vi "Const Lang Default English.vi"() -> (3 "UI Descriptions":T1={"Main Panel"={"Title"={"Frame Num"={"Name"="Frame Num", "Tip"="", "Description"=""}, "Name"={"Name"="Name", "Tip"="", "Description"=""}}, "Frame Basic"={"pic"={"Name"="pic", "Tip"="", "Description"=""}, "state"={"Name"="state", "Tip"="", "Description"=""}, "wait"={"Name"="wait", "Tip"="", "Description"=""}, "next"={"Name"="next", "Tip"="Next frame number", "Description"="Next frame number  \n999: Return to frame number 0  \n1000: Remove object  \n12XX: Invisible, where XX represents the duration  \nA minus sign indicates direction reversal"}, "dvx"={"Name"="dvx", "Tip"="movement speed", "Description"="Forward (positive) and backward (negative) movement speed"}, "dvy"={"Name"="dvy", "Tip"="movement speed", "Description"="Upward (negative) and downward (positive) movement speed"}, "dvz"={"Name"="dvz", "Tip"="movement speed", "Description"="Vertical movement speed, with the direction determined by the ◆ and □ arrow keys"}, "centerx"={"Name"="centerx", "Tip"="X-axis position of the frame center", "Description"="X-axis position of the frame center (shadow), with direction from left to right"}, "centery"={"Name"="centery", "Tip"="Y-axis position of the frame center", "Description"="Y-axis position of the frame center (shadow), with direction from top to bottom"}, "sound"={"Name"="sound", "Tip"="", "Description"=""}}, "Frame Skill"={"mp"={"Name"="mp", "Tip"="HP/MP Consumption", "Description"="HP/MP Consumption  \nOOXXX: OO represents the tens digit of HP consumption, XXX represents MP consumption  \n100: Consumes 100 MP  \n4300: Consumes 40 HP and 300 MP  \n\nWhen entering a frame using hit_XX:  \n  - Positive values indicate consumption  \n  - Negative values indicate recovery  \n\nWhen entering a frame using next:  \n  - Positive values have no effect  \n  - Negative values indicate consumption"}, "hit_a"={"Name"="hit_a", "Tip"="When pressing Attack, jump to the corresponding frame number", "Description"="When pressing Attack, jump to the corresponding frame number"}, "hit_d"={"Name"="hit_d", "Tip"="When pressing Defense, jump to the corresponding frame number", "Description"="When pressing Defense, jump to the corresponding frame number"}, "hit_j"={"Name"="hit_j", "Tip"="When pressing Jump, jump to the corresponding frame number", "Description"="When pressing Jump, jump to the corresponding frame number"}, "hit_Fa"={"Name"="hit_Fa", "Tip"="When pressing Defense △ Attack, jump to the corresponding frame number", "Description"="When pressing Defense △ Attack, jump to the corresponding frame number"}, "hit_Ua"={"Name"="hit_Ua", "Tip"="When pressing Defense ◆ Attack, jump to the corresponding frame number", "Description"="When pressing Defense ◆ Attack, jump to the corresponding frame number"}, "hit_Da"={"Name"="hit_Da", "Tip"="When pressing Defense □ Attack, jump to the corresponding frame number", "Description"="When pressing Defense □ Attack, jump to the corresponding frame number"}, "hit_Fj"={"Name"="hit_Fj", "Tip"="When pressing Defense △ Jump, jump to the corresponding frame number", "Description"="When pressing Defense △ Jump, jump to the corresponding frame number"}, "hit_Uj"={"Name"="hit_Uj", "Tip"="When pressing Defense ◆ Jump, jump to the corresponding frame number", "Description"="When pressing Defense ◆ Jump, jump to the corresponding frame number"}, "hit_Dj"={"Name"="hit_Dj", "Tip"="When pressing Defense □ Jump, jump to the corresponding frame number", "Description"="When pressing Defense □ Jump, jump to the corresponding frame number"}, "hit_ja"={"Name"="hit_ja", "Tip"="When pressing Defense + Jump + Attack, jump to the corresponding frame number", "Description"="When pressing Defense + Jump + Attack, jump to the corresponding frame number"}}, "bp"={"x"={"Name"="x", "Tip"="X-axis position of mouth bleeding", "Description"="X-axis position of mouth bleeding\nBleeding occurs when HP is less than 1/3"}, "y"={"Name"="y", "Tip"="Y-axis position of mouth bleeding", "Description"="Y-axis position of mouth bleeding\nBleeding occurs when HP is less than 1/3"}}, "w"={"kind"={"Name"="kind", "Tip"="Weapon state\n1: Held in hand  \n2: Held in hand  \n3: Dropped", "Description"="Weapon state\n1: Held in hand  \n2: Held in hand  \n3: Dropped"}, "x"={"Name"="x", "Tip"="X-axis position of the weapon", "Description"="X-axis position of the weapon"}, "y"={"Name"="y", "Tip"="Y-axis position of the weapon", "Description"="Y-axis position of the weapon"}, "weaponact"={"Name"="weaponact", "Tip"="Weapon frame number\nIf outside 20~35, the weapon can be hit", "Description"="Weapon frame number\nIf outside 20~35, the weapon can be hit"}, "cover"={"Name"="cover", "Tip"="0: Weapon in front (overlays the character image)  \n1: Weapon behind (character overlays the weapon image)", "Description"="0: Weapon in front (overlays the character image)  \n1: Weapon behind (character overlays the weapon image)"}, "dvx"={"Name"="dvx", "Tip"="movement speed", "Description"="Forward (positive) and backward (negative) movement speed"}, "dvy"={"Name"="dvy", "Tip"="movement speed", "Description"="Upward (negative) and downward (positive) movement speed"}, "dvz"={"Name"="dvz", "Tip"="movement speed", "Description"="Vertical movement speed, with the direction determined by the ◆ and □ arrow keys"}, "attacking"={"Name"="attacking", "Tip"="Attack state", "Description"="Attack state\n0: No attack  \n1: Attack while standing  \n2: Attack while jumping  \n3: Attack while running  \n4: Attack while jumping forward"}}, "b"={"kind"={"Name"="kind", "Tip"="", "Description"=""}, "x"={"Name"="x", "Tip"="X-axis position of the hitbox", "Description"="X-axis position of the hitbox"}, "y"={"Name"="y", "Tip"="Y-axis position of the hitbox", "Description"="Y-axis position of the hitbox"}, "w"={"Name"="w", "Tip"="Width of the hitbox", "Description"="Width of the hitbox"}, "h"={"Name"="h", "Tip"="Height of the hitbox", "Description"="Height of the hitbox"}, "index"={"Name"="<b> index", "Tip"="body section index", "Description"="body section index"}}, "i"={"kind"={"Name"="kind", "Tip"="Injury Effect", "Description"="Injury Effect\n0: Normal attack / effect attack  \n1: Grab a stunned opponent (state 16)  \n2: Pick up a weapon  \n3: Forced grab  \n4: Attack type when thrown by an enemy  \n5: Weapon type  \n6: If an enemy is within this range, jump to a super_punch frame  \n7: Press Attack to pick up a weapon immediately  \n8: Convert injury to healing, jump to dvx frame  \n9: Reduce HP to zero after hitting an enemy  \n10: Henry's \"Death Symphony\" effect  \n11: Henry's \"Death Symphony\" effect  \n14: Block  \n15: Float  \n16: Freeze"}, "x"={"Name"="x", "Tip"="X-axis position of the hitbox", "Description"="X-axis position of the hitbox"}, "y"={"Name"="y", "Tip"="Y-axis position of the hitbox", "Description"="Y-axis position of the hitbox"}, "w"={"Name"="w", "Tip"="Width of the hitbox", "Description"="Width of the hitbox"}, "h"={"Name"="h", "Tip"="Height of the hitbox", "Description"="Height of the hitbox"}, "zwidth"={"Name"="zwidth", "Tip"="Width of the hitbox along the Z-axis", "Description"="Width of the hitbox along the Z-axis"}, "dvx"={"Name"="dvx", "Tip"="movement speed", "Description"="Forward (positive) and backward (negative) movement speed"}, "dvy"={"Name"="dvy", "Tip"="movement speed", "Description"="Upward (negative) and downward (positive) movement speed"}, "dvz"={"Name"="dvz", "Tip"="movement speed", "Description"="Vertical movement speed, with the direction determined by the ◆ and □ arrow keys"}, "fall"={"Name"="fall", "Tip"="Knockdown value", "Description"="Knockdown value\n1: Enemy pauses briefly, but the value does not accumulate toward stun  \n25: Hitting twice will stun the enemy  \n40: First hit makes the enemy step back, second hit knocks them down  \n60: First hit stuns the enemy, second hit knocks them down  \n70: Forced knockdown  \nNegative value: Does not affect the enemy's action, but grants super armor (enemy shows no hurt animation)"}, "arest"={"Name"="arest", "Tip"="Interval for repeatedly attacking a single enemy\nForcibly disables vrest", "Description"="Interval for repeatedly attacking a single enemy\nForcibly disables vrest"}, "vrest"={"Name"="vrest", "Tip"="Interval for repeatedly attacking multiple enemies\nCannot be used simultaneously with arest\nMinimum value is 4", "Description"="Interval for repeatedly attacking multiple enemies\nCannot be used simultaneously with arest\nMinimum value is 4"}, "bdefend"={"Name"="bdefend", "Tip"="Guard break value", "Description"="Guard break value\nAccumulate up to 60 to break a defending enemy  \n60: Directly breaks guard  \n100: Ignores all defense and hits directly. Items are forcibly destroyed"}, "injury"={"Name"="injury", "Tip"="", "Description"=""}, "effect"={"Name"="effect", "Tip"="Attack special effect (only for kind:0)", "Description"="Attack special effect (only for kind:0)\n0: Fist effect  \n1: Bladed weapon effect  \n2: Fire  \n20: Fire, cannot hit ball attacks  \n21: Fire, can reflect ball attacks; when combined with state 18 (fire), it will not hit allies  \n22: Fire; if dvx is positive, attack direction is inward; if dvx is negative, attack direction is outward  \n23: Hit effect; if dvx is positive, attack direction is inward; if dvx is negative, attack direction is outward  \n3: Freeze  \n30: Freeze; cannot hit state 13 characters (frozen characters)  \n4: Only attacks objects of type: 1, 2, 3, 4, 5, 6"}, "catchingact 1"={"Name"="catchingact 1", "Tip"="Only for kind: 1 (grab stunned enemy), kind: 3 (forced grab)\nAfter grabbing an enemy, jumps to the frame number", "Description"="Only for kind: 1 (grab stunned enemy), kind: 3 (forced grab)\nAfter grabbing an enemy, jumps to the frame number"}, "catchingact 2"={"Name"="catchingact 2", "Tip"="Only for kind: 1 (grab stunned enemy), kind: 3 (forced grab)\nAfter grabbing an enemy, jumps to the frame number", "Description"="Only for kind: 1 (grab stunned enemy), kind: 3 (forced grab)\nAfter grabbing an enemy, jumps to the frame number"}, "caughtact 1"={"Name"="caughtact 1", "Tip"="Only for kind: 1 (grab stunned enemy), kind: 3 (forced grab)\nAfter grabbing an enemy, the enemy's frame number jumps to the frame number", "Description"="Only for kind: 1 (grab stunned enemy), kind: 3 (forced grab)\nAfter grabbing an enemy, jumps to the frame number"}, "caughtact 2"={"Name"="caughtact 2", "Tip"="Only for kind: 1 (grab stunned enemy), kind: 3 (forced grab)\nAfter grabbing an enemy, the enemy's frame number jumps to the frame number", "Description"="Only for kind: 1 (grab stunned enemy), kind: 3 (forced grab)\nAfter grabbing an enemy, the enemy's frame number jumps to the frame number"}, "index"={"Name"="<i> index", "Tip"="injury section index", "Description"="injury section index"}}, "o"={"kind"={"Name"="kind", "Tip"="Creation type", "Description"="Creation type\n1: Dropped  \n2: Held in hand"}, "x"={"Name"="x", "Tip"="X-axis position of the object, with direction from left to right", "Description"="X-axis position of the object, with direction from left to right"}, "y"={"Name"="y", "Tip"="Y-axis position of the object, with direction from top to bottom", "Description"="Y-axis position of the object, with direction from top to bottom"}, "action"={"Name"="action", "Tip"="Frame number of the object", "Description"="Frame number of the object"}, "dvx"={"Name"="dvx", "Tip"="movement speed", "Description"="Forward (positive) and backward (negative) movement speed of the object"}, "dvy"={"Name"="dvy", "Tip"="movement speed", "Description"="Upward (negative) and downward (positive) movement speed of the object"}, "dvz"={"Name"="dvz", "Tip"="movement speed", "Description"="Vertical movement speed of the object, with direction determined by the ◆ and □ arrow keys"}, "oid"={"Name"="oid", "Tip"="Object ID", "Description"="Object ID"}, "facing"={"Name"="facing", "Tip"="Object quantity and direction", "Description"="Object quantity and direction\nOOX: OO represents the quantity. X represents the direction, where 0 = forward, 1 = reverse"}}, "c"={"kind"={"Name"="kind", "Tip"="Grab state", "Description"="1: Grabber  \n2: Grabbed"}, "x"={"Name"="x", "Tip"="X-axis position of the grabber/grabbed", "Description"="X-axis position of the grabber/grabbed"}, "y"={"Name"="y", "Tip"="Y-axis position of the grabber/grabbed", "Description"="Y-axis position of the grabber/grabbed"}, "injury"={"Name"="injury", "Tip"="Damage\nPositive value: Causes injury with hit pause effect  \nNegative value: Causes injury without hit pause effect", "Description"="Damage\nPositive value: Causes injury with hit pause effect  \nNegative value: Causes injury without hit pause effect"}, "cover"={"Name"="cover", "Tip"="Layer order\n10: Grabbed character behind  \n11: Grabbed character in front", "Description"="Layer order\n10: Grabbed character behind  \n11: Grabbed character in front"}, "vaction"={"Name"="vaction", "Tip"="Frame number of the grabbed character", "Description"="Frame number of the grabbed character"}, "aaction"={"Name"="aaction", "Tip"="When pressing Attack, jump to the corresponding frame number", "Description"="When pressing Attack, jump to the corresponding frame number"}, "taction"={"Name"="taction", "Tip"="When pressing △ + Attack, jump to the corresponding frame number", "Description"="When pressing △ + Attack, jump to the corresponding frame number"}, "hurtable"={"Name"="hurtable", "Tip"="Whether the grabbed character can be hit by others\n0: No  \n1: Yes", "Description"="Whether the grabbed character can be hit by others\n0: No  \n1: Yes"}, "decrease"={"Name"="decrease", "Tip"="Decrement value for grab duration (negative value), total duration is 301", "Description"="Decrement value for grab duration (negative value), total duration is 301"}, "fronthurtact"={"Name"="fronthurtact", "Tip"="Jump to Frame number after being hit from the front", "Description"="Jump to Frame number after being hit from the front"}, "backhurtact"={"Name"="backhurtact", "Tip"="Jump to Frame number after being hit from the back", "Description"="Jump to Frame number after being hit from the back"}, "throwvx"={"Name"="throwvx", "Tip"="X-direction speed when thrown", "Description"="X-direction speed when thrown"}, "throwvy"={"Name"="throwvy", "Tip"="Y-direction speed when thrown", "Description"="Y-direction speed when thrown"}, "throwvz"={"Name"="throwvz", "Tip"="Z-direction speed when thrown, with direction determined by the ◆ and □ arrow keys", "Description"="Z-direction speed when thrown, with direction determined by the ◆ and □ arrow keys"}, "throwinjury"={"Name"="throwinjury", "Tip"="", "Description"=""}, "dircontrol"={"Name"="dircontrol", "Tip"="", "Description"=""}}, "Other"={"File Path"={"Name"="File Path", "Tip"="", "Description"=""}, "GoTo"={"Name"="Go to Frame", "Tip"="", "Description"=""}, "Apply Change"={"Name"="Apply Change", "Tip"="", "Description"=""}, "To Next Frame"={"Name"="To Next Frame", "Tip"="", "Description"=""}}, "Menu"={"File"={"Name"="File", "Tip"="", "Description"=""}, "Open File"={"Name"="Open File", "Tip"="", "Description"=""}, "Save File"={"Name"="Save File", "Tip"="", "Description"=""}, "Exit"={"Name"="Exit", "Tip"="", "Description"=""}, "Settings"={"Name"="Settings", "Tip"="", "Description"=""}, "Preferences"={"Name"="Preferences", "Tip"="", "Description"=""}, "Help"={"Name"="Help", "Tip"="", "Description"=""}, "Show Context Help"={"Name"="Show Context Help", "Tip"="", "Description"=""}}}, "Configuration Window"={"Tab"={"Main Page"={"Name"="Main", "Tip"="", "Description"=""}, "Image Page"={"Name"="Image", "Tip"="", "Description"=""}}, "Main"={"Language"={"Name"="Language", "Tip"="", "Description"=""}, "Save"={"Name"="Save", "Tip"="", "Description"=""}, "Cancel"={"Name"="Cancel", "Tip"="", "Description"=""}}, "Path"={"Reset"={"Name"="Reset to Steam Path", "Tip"="", "Description"=""}, "Path Data"={"Name"="_res_data Folder Path", "Tip"="", "Description"=""}, "Path Png"={"Name"="_res_pngs Folder Path", "Tip"="", "Description"=""}}, "Image"={"Center Point"={"Name"={"Name"="Center Point:", "Tip"="", "Description"=""}, "Size"={"Name"="Size", "Tip"="", "Description"=""}, "Color"={"Name"="Color", "Tip"="", "Description"=""}, "Enable"={"Name"="Enable", "Tip"="", "Description"=""}}, "bp Point"={"Name"={"Name"="<bp> Point:", "Tip"="", "Description"=""}, "Size"={"Name"="Size", "Tip"="", "Description"=""}, "Color"={"Name"="Color", "Tip"="", "Description"=""}, "Enable"={"Name"="Enable", "Tip"="", "Description"=""}}, "w Point"={"Name"={"Name"="<w> Point:", "Tip"="", "Description"=""}, "Size"={"Name"="Size", "Tip"="", "Description"=""}, "Color"={"Name"="Color", "Tip"="", "Description"=""}, "Enable"={"Name"="Enable", "Tip"="", "Description"=""}}, "b Box"={"Name"={"Name"="<b> Box:", "Tip"="", "Description"=""}, "Fill Color"={"Name"="Fill Color", "Tip"="", "Description"=""}, "Border Color"={"Name"="Border Color", "Tip"="", "Description"=""}, "Enable"={"Name"="Enable", "Tip"="", "Description"=""}}, "i Box"={"Name"={"Name"="<i> Box:", "Tip"="", "Description"=""}, "Fill Color"={"Name"="Fill Color", "Tip"="", "Description"=""}, "Border Color"={"Name"="Border Color", "Tip"="", "Description"=""}, "Enable"={"Name"="Enable", "Tip"="", "Description"=""}}, "o Point"={"Name"={"Name"="<o> Point:", "Tip"="", "Description"=""}, "Size"={"Name"="Size", "Tip"="", "Description"=""}, "Color"={"Name"="Color", "Tip"="", "Description"=""}, "Enable"={"Name"="Enable", "Tip"="", "Description"=""}}, "c Point"={"Name"={"Name"="<c> Point:", "Tip"="", "Description"=""}, "Size"={"Name"="Size", "Tip"="", "Description"=""}, "Color"={"Name"="Color", "Tip"="", "Description"=""}, "Enable"={"Name"="Enable", "Tip"="", "Description"=""}}}}})   [LabVIEW 2018, in "Framework.lvlib" / "Framework.lvclass"]
uses:
  Framework/Framework/Framework.lvclass
  Const Lang Setting.ctl
  Const UI Desc Frame Title.ctl
  Const Lang Property.ctl
  Const UI Desc Frame Basic.ctl
  Const UI Desc Frame Skill.ctl
  Const UI Desc Frame bp.ctl
  Const UI Desc Frame w.ctl
  Const UI Desc Frame b.ctl
  Const UI Desc Frame i.ctl
  Const UI Desc Frame o.ctl
  Const UI Desc Frame c.ctl
  Const UI Desc Other.ctl
  Const UI Desc Menu.ctl
  Const Lang CfgWnd Tab.ctl
  Const Lang CfgWnd Main.ctl
  Const Lang CfgWnd Path.ctl
  Framework/Framework/Const Lang CfgWnd Image.ctl
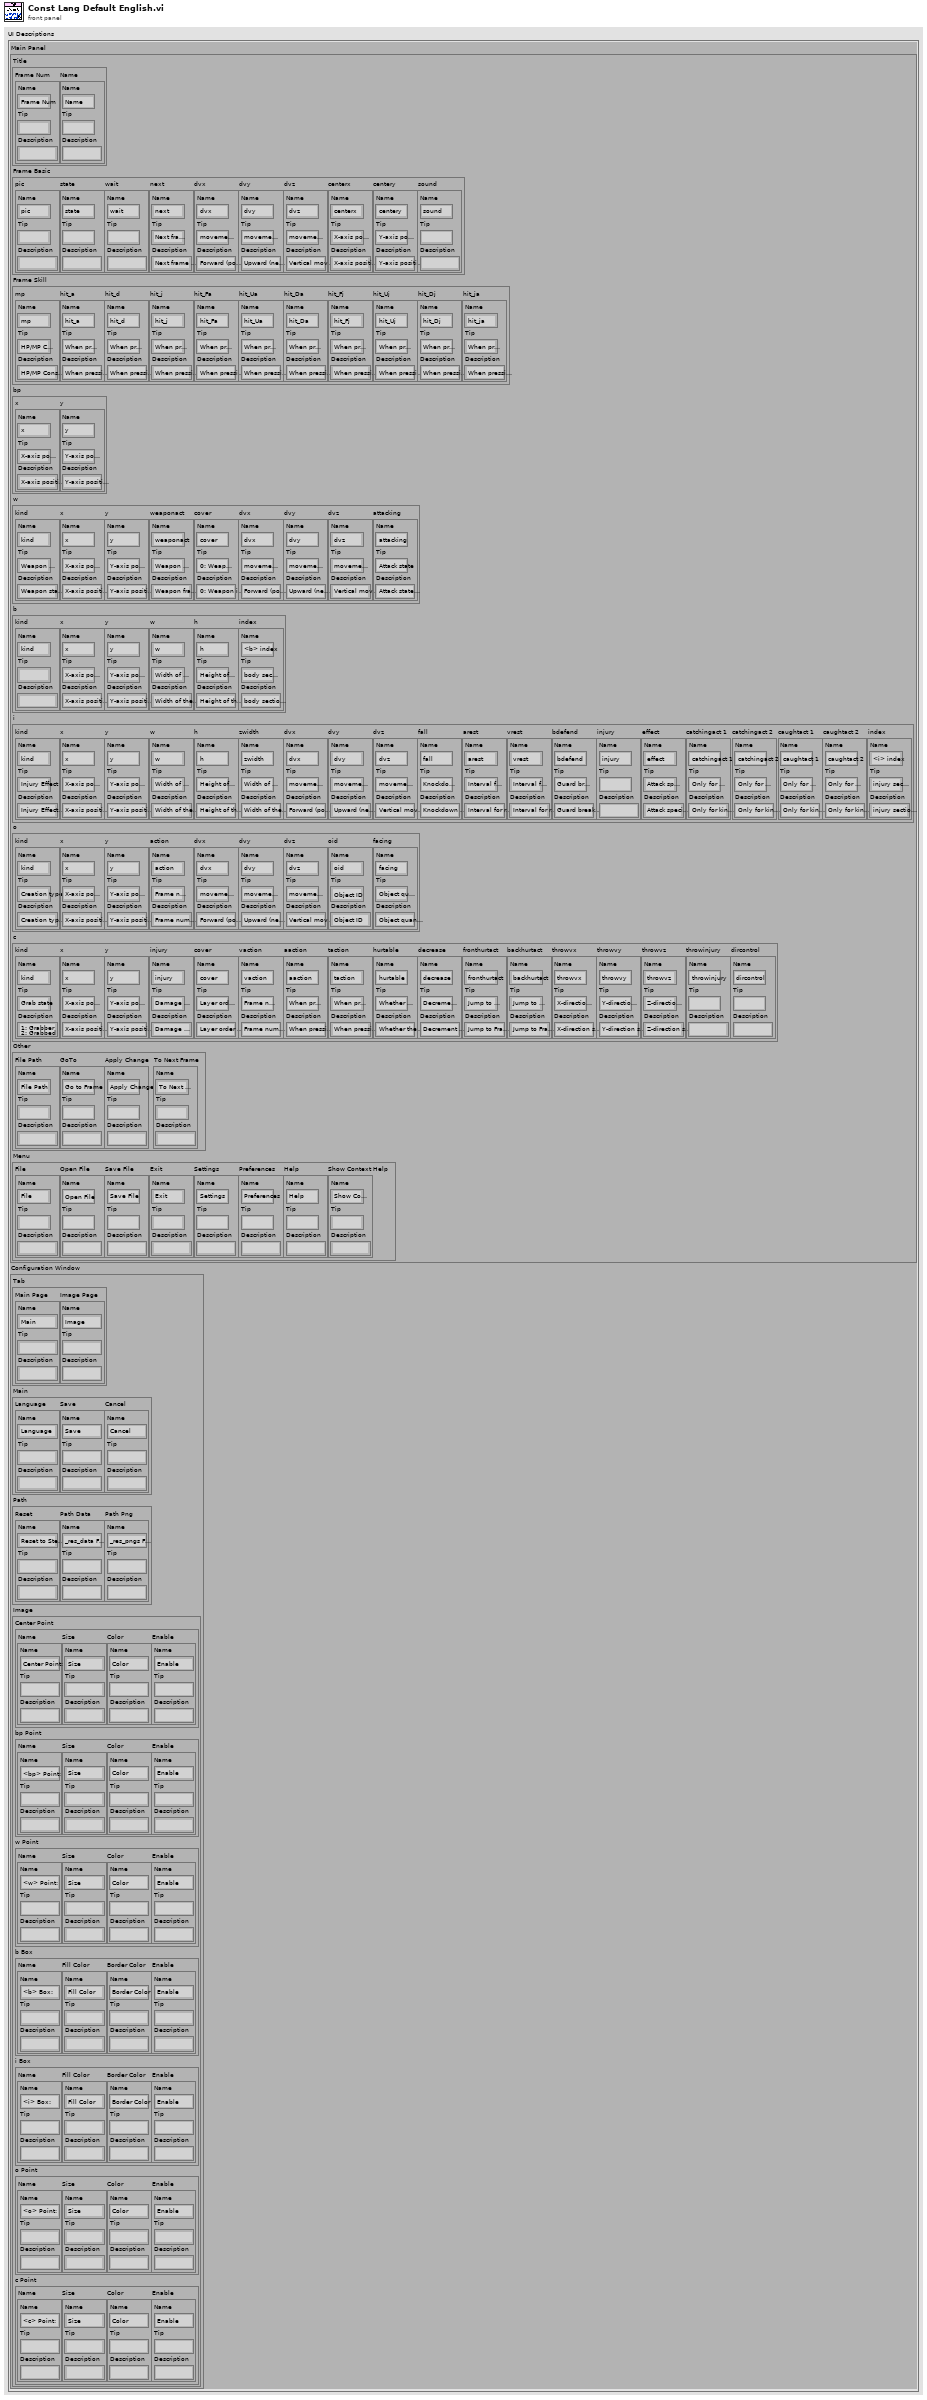
[diagram p1: front panel]
types:
  T1 = typedef "Framework.lvlib/Framework.lvclass/Const Lang Setting.ctl" = cluster{"Main Panel":cluster{"Title":T2, "Frame Basic":T4, "Frame Skill":T5, "bp":T6, "w":T7, "b":T8, "i":T9, "o":T10, "c":T11, "Other":T12, "Menu":T13}, "Configuration Window":cluster{"Tab":T14, "Main":T15, "Path":T16, "Image":T17}}
  T2 = typedef "Framework.lvlib/Framework.lvclass/Const UI Desc Frame Title.ctl" = cluster{"Frame Num":T3, "Name":T3}
  T3 = typedef "Framework.lvlib/Framework.lvclass/Const Lang Property.ctl" = cluster{"Name":string, "Tip":string, "Description":string}
  T4 = typedef "Framework.lvlib/Framework.lvclass/Const UI Desc Frame Basic.ctl" = cluster{"pic":T3, "state":T3, "wait":T3, "next":T3, "dvx":T3, "dvy":T3, "dvz":T3, "centerx":T3, "centery":T3, "sound":T3}
  T5 = typedef "Framework.lvlib/Framework.lvclass/Const UI Desc Frame Skill.ctl" = cluster{"mp":T3, "hit_a":T3, "hit_d":T3, "hit_j":T3, "hit_Fa":T3, "hit_Ua":T3, "hit_Da":T3, "hit_Fj":T3, "hit_Uj":T3, "hit_Dj":T3, "hit_ja":T3}
  T6 = typedef "Framework.lvlib/Framework.lvclass/Const UI Desc Frame bp.ctl" = cluster{"x":T3, "y":T3}
  T7 = typedef "Framework.lvlib/Framework.lvclass/Const UI Desc Frame w.ctl" = cluster{"kind":T3, "x":T3, "y":T3, "weaponact":T3, "cover":T3, "dvx":T3, "dvy":T3, "dvz":T3, "attacking":T3}
  T8 = typedef "Framework.lvlib/Framework.lvclass/Const UI Desc Frame b.ctl" = cluster{"kind":T3, "x":T3, "y":T3, "w":T3, "h":T3, "index":T3}
  T9 = typedef "Framework.lvlib/Framework.lvclass/Const UI Desc Frame i.ctl" = cluster{"kind":T3, "x":T3, "y":T3, "w":T3, "h":T3, "zwidth":T3, "dvx":T3, "dvy":T3, "dvz":T3, "fall":T3, "arest":T3, "vrest":T3, "bdefend":T3, "injury":T3, "effect":T3, "catchingact 1":T3, "catchingact 2":T3, "caughtact 1":T3, "caughtact 2":T3, "index":T3}
  T10 = typedef "Framework.lvlib/Framework.lvclass/Const UI Desc Frame o.ctl" = cluster{"kind":T3, "x":T3, "y":T3, "action":T3, "dvx":T3, "dvy":T3, "dvz":T3, "oid":T3, "facing":T3}
  T11 = typedef "Framework.lvlib/Framework.lvclass/Const UI Desc Frame c.ctl" = cluster{"kind":T3, "x":T3, "y":T3, "injury":T3, "cover":T3, "vaction":T3, "aaction":T3, "taction":T3, "hurtable":T3, "decrease":T3, "fronthurtact":T3, "backhurtact":T3, "throwvx":T3, "throwvy":T3, "throwvz":T3, "throwinjury":T3, "dircontrol":T3}
  T12 = typedef "Framework.lvlib/Framework.lvclass/Const UI Desc Other.ctl" = cluster{"File Path":T3, "GoTo":T3, "Apply Change":T3, "To Next Frame":T3}
  T13 = typedef "Framework.lvlib/Framework.lvclass/Const UI Desc Menu.ctl" = cluster{"File":T3, "Open File":T3, "Save File":T3, "Exit":T3, "Settings":T3, "Preferences":T3, "Help":T3, "Show Context Help":T3}
  T14 = typedef "Framework.lvlib/Framework.lvclass/Const Lang CfgWnd Tab.ctl" = cluster{"Main Page":T3, "Image Page":T3}
  T15 = typedef "Framework.lvlib/Framework.lvclass/Const Lang CfgWnd Main.ctl" = cluster{"Language":T3, "Save":T3, "Cancel":T3}
  T16 = typedef "Framework.lvlib/Framework.lvclass/Const Lang CfgWnd Path.ctl" = cluster{"Reset":T3, "Path Data":T3, "Path Png":T3}
  T17 = typedef "Framework.lvlib/Framework.lvclass/Const Lang CfgWnd Image.ctl" = cluster{"Center Point":cluster{"Name":T3, "Size":T3, "Color":T3, "Enable":T3}, "bp Point":cluster{"Name":T3, "Size":T3, "Color":T3, "Enable":T3}, "w Point":cluster{"Name":T3, "Size":T3, "Color":T3, "Enable":T3}, "b Box":cluster{"Name":T3, "Fill Color":T3, "Border Color":T3, "Enable":T3}, "i Box":cluster{"Name":T3, "Fill Color":T3, "Border Color":T3, "Enable":T3}, "o Point":cluster{"Name":T3, "Size":T3, "Color":T3, "Enable":T3}, "c Point":cluster{"Name":T3, "Size":T3, "Color":T3, "Enable":T3}}
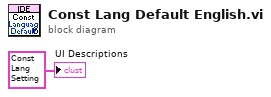
[diagram p0: block diagram]
diagram:
  "UI Descriptions" <- T1 {"Main Panel"={"Title"={"Frame Num"={"Name"="Frame Num", "Tip"="", "Description"=""}, "Name"={"Name"="Name", "Tip"="", "Description"=""}}, "Frame Basic"={"pic"={"Name"="pic", "Tip"="", "Description"=""}, "state"={"Name"="state", "Tip"="", "Description"=""}, "wait"={"Name"="wait", "Tip"="", "Description"=""}, "next"={"Name"="next", "Tip"="Next frame number", "Description"="Next frame number  \n999: Return to frame number 0  \n1000: Remove object  \n12XX: Invisible, where XX represents the duration  \nA minus sign indicates direction reversal"}, "dvx"={"Name"="dvx", "Tip"="movement speed", "Description"="Forward (positive) and backward (negative) movement speed"}, "dvy"={"Name"="dvy", "Tip"="movement speed", "Description"="Upward (negative) and downward (positive) movement speed"}, "dvz"={"Name"="dvz", "Tip"="movement speed", "Description"="Vertical movement speed, with the direction determined by the ◆ and □ arrow keys"}, "centerx"={"Name"="centerx", "Tip"="X-axis position of the frame center", "Description"="X-axis position of the frame center (shadow), with direction from left to right"}, "centery"={"Name"="centery", "Tip"="Y-axis position of the frame center", "Description"="Y-axis position of the frame center (shadow), with direction from top to bottom"}, "sound"={"Name"="sound", "Tip"="", "Description"=""}}, "Frame Skill"={"mp"={"Name"="mp", "Tip"="HP/MP Consumption", "Description"="HP/MP Consumption  \nOOXXX: OO represents the tens digit of HP consumption, XXX represents MP consumption  \n100: Consumes 100 MP  \n4300: Consumes 40 HP and 300 MP  \n\nWhen entering a frame using hit_XX:  \n  - Positive values indicate consumption  \n  - Negative values indicate recovery  \n\nWhen entering a frame using next:  \n  - Positive values have no effect  \n  - Negative values indicate consumption"}, "hit_a"={"Name"="hit_a", "Tip"="When pressing Attack, jump to the corresponding frame number", "Description"="When pressing Attack, jump to the corresponding frame number"}, "hit_d"={"Name"="hit_d", "Tip"="When pressing Defense, jump to the corresponding frame number", "Description"="When pressing Defense, jump to the corresponding frame number"}, "hit_j"={"Name"="hit_j", "Tip"="When pressing Jump, jump to the corresponding frame number", "Description"="When pressing Jump, jump to the corresponding frame number"}, "hit_Fa"={"Name"="hit_Fa", "Tip"="When pressing Defense △ Attack, jump to the corresponding frame number", "Description"="When pressing Defense △ Attack, jump to the corresponding frame number"}, "hit_Ua"={"Name"="hit_Ua", "Tip"="When pressing Defense ◆ Attack, jump to the corresponding frame number", "Description"="When pressing Defense ◆ Attack, jump to the corresponding frame number"}, "hit_Da"={"Name"="hit_Da", "Tip"="When pressing Defense □ Attack, jump to the corresponding frame number", "Description"="When pressing Defense □ Attack, jump to the corresponding frame number"}, "hit_Fj"={"Name"="hit_Fj", "Tip"="When pressing Defense △ Jump, jump to the corresponding frame number", "Description"="When pressing Defense △ Jump, jump to the corresponding frame number"}, "hit_Uj"={"Name"="hit_Uj", "Tip"="When pressing Defense ◆ Jump, jump to the corresponding frame number", "Description"="When pressing Defense ◆ Jump, jump to the corresponding frame number"}, "hit_Dj"={"Name"="hit_Dj", "Tip"="When pressing Defense □ Jump, jump to the corresponding frame number", "Description"="When pressing Defense □ Jump, jump to the corresponding frame number"}, "hit_ja"={"Name"="hit_ja", "Tip"="When pressing Defense + Jump + Attack, jump to the corresponding frame number", "Description"="When pressing Defense + Jump + Attack, jump to the corresponding frame number"}}, "bp"={"x"={"Name"="x", "Tip"="X-axis position of mouth bleeding", "Description"="X-axis position of mouth bleeding\nBleeding occurs when HP is less than 1/3"}, "y"={"Name"="y", "Tip"="Y-axis position of mouth bleeding", "Description"="Y-axis position of mouth bleeding\nBleeding occurs when HP is less than 1/3"}}, "w"={"kind"={"Name"="kind", "Tip"="Weapon state\n1: Held in hand  \n2: Held in hand  \n3: Dropped", "Description"="Weapon state\n1: Held in hand  \n2: Held in hand  \n3: Dropped"}, "x"={"Name"="x", "Tip"="X-axis position of the weapon", "Description"="X-axis position of the weapon"}, "y"={"Name"="y", "Tip"="Y-axis position of the weapon", "Description"="Y-axis position of the weapon"}, "weaponact"={"Name"="weaponact", "Tip"="Weapon frame number\nIf outside 20~35, the weapon can be hit", "Description"="Weapon frame number\nIf outside 20~35, the weapon can be hit"}, "cover"={"Name"="cover", "Tip"="0: Weapon in front (overlays the character image)  \n1: Weapon behind (character overlays the weapon image)", "Description"="0: Weapon in front (overlays the character image)  \n1: Weapon behind (character overlays the weapon image)"}, "dvx"={"Name"="dvx", "Tip"="movement speed", "Description"="Forward (positive) and backward (negative) movement speed"}, "dvy"={"Name"="dvy", "Tip"="movement speed", "Description"="Upward (negative) and downward (positive) movement speed"}, "dvz"={"Name"="dvz", "Tip"="movement speed", "Description"="Vertical movement speed, with the direction determined by the ◆ and □ arrow keys"}, "attacking"={"Name"="attacking", "Tip"="Attack state", "Description"="Attack state\n0: No attack  \n1: Attack while standing  \n2: Attack while jumping  \n3: Attack while running  \n4: Attack while jumping forward"}}, "b"={"kind"={"Name"="kind", "Tip"="", "Description"=""}, "x"={"Name"="x", "Tip"="X-axis position of the hitbox", "Description"="X-axis position of the hitbox"}, "y"={"Name"="y", "Tip"="Y-axis position of the hitbox", "Description"="Y-axis position of the hitbox"}, "w"={"Name"="w", "Tip"="Width of the hitbox", "Description"="Width of the hitbox"}, "h"={"Name"="h", "Tip"="Height of the hitbox", "Description"="Height of the hitbox"}, "index"={"Name"="<b> index", "Tip"="body section index", "Description"="body section index"}}, "i"={"kind"={"Name"="kind", "Tip"="Injury Effect", "Description"="Injury Effect\n0: Normal attack / effect attack  \n1: Grab a stunned opponent (state 16)  \n2: Pick up a weapon  \n3: Forced grab  \n4: Attack type when thrown by an enemy  \n5: Weapon type  \n6: If an enemy is within this range, jump to a super_punch frame  \n7: Press Attack to pick up a weapon immediately  \n8: Convert injury to healing, jump to dvx frame  \n9: Reduce HP to zero after hitting an enemy  \n10: Henry's \"Death Symphony\" effect  \n11: Henry's \"Death Symphony\" effect  \n14: Block  \n15: Float  \n16: Freeze"}, "x"={"Name"="x", "Tip"="X-axis position of the hitbox", "Description"="X-axis position of the hitbox"}, "y"={"Name"="y", "Tip"="Y-axis position of the hitbox", "Description"="Y-axis position of the hitbox"}, "w"={"Name"="w", "Tip"="Width of the hitbox", "Description"="Width of the hitbox"}, "h"={"Name"="h", "Tip"="Height of the hitbox", "Description"="Height of the hitbox"}, "zwidth"={"Name"="zwidth", "Tip"="Width of the hitbox along the Z-axis", "Description"="Width of the hitbox along the Z-axis"}, "dvx"={"Name"="dvx", "Tip"="movement speed", "Description"="Forward (positive) and backward (negative) movement speed"}, "dvy"={"Name"="dvy", "Tip"="movement speed", "Description"="Upward (negative) and downward (positive) movement speed"}, "dvz"={"Name"="dvz", "Tip"="movement speed", "Description"="Vertical movement speed, with the direction determined by the ◆ and □ arrow keys"}, "fall"={"Name"="fall", "Tip"="Knockdown value", "Description"="Knockdown value\n1: Enemy pauses briefly, but the value does not accumulate toward stun  \n25: Hitting twice will stun the enemy  \n40: First hit makes the enemy step back, second hit knocks them down  \n60: First hit stuns the enemy, second hit knocks them down  \n70: Forced knockdown  \nNegative value: Does not affect the enemy's action, but grants super armor (enemy shows no hurt animation)"}, "arest"={"Name"="arest", "Tip"="Interval for repeatedly attacking a single enemy\nForcibly disables vrest", "Description"="Interval for repeatedly attacking a single enemy\nForcibly disables vrest"}, "vrest"={"Name"="vrest", "Tip"="Interval for repeatedly attacking multiple enemies\nCannot be used simultaneously with arest\nMinimum value is 4", "Description"="Interval for repeatedly attacking multiple enemies\nCannot be used simultaneously with arest\nMinimum value is 4"}, "bdefend"={"Name"="bdefend", "Tip"="Guard break value", "Description"="Guard break value\nAccumulate up to 60 to break a defending enemy  \n60: Directly breaks guard  \n100: Ignores all defense and hits directly. Items are forcibly destroyed"}, "injury"={"Name"="injury", "Tip"="", "Description"=""}, "effect"={"Name"="effect", "Tip"="Attack special effect (only for kind:0)", "Description"="Attack special effect (only for kind:0)\n0: Fist effect  \n1: Bladed weapon effect  \n2: Fire  \n20: Fire, cannot hit ball attacks  \n21: Fire, can reflect ball attacks; when combined with state 18 (fire), it will not hit allies  \n22: Fire; if dvx is positive, attack direction is inward; if dvx is negative, attack direction is outward  \n23: Hit effect; if dvx is positive, attack direction is inward; if dvx is negative, attack direction is outward  \n3: Freeze  \n30: Freeze; cannot hit state 13 characters (frozen characters)  \n4: Only attacks objects of type: 1, 2, 3, 4, 5, 6"}, "catchingact 1"={"Name"="catchingact 1", "Tip"="Only for kind: 1 (grab stunned enemy), kind: 3 (forced grab)\nAfter grabbing an enemy, jumps to the frame number", "Description"="Only for kind: 1 (grab stunned enemy), kind: 3 (forced grab)\nAfter grabbing an enemy, jumps to the frame number"}, "catchingact 2"={"Name"="catchingact 2", "Tip"="Only for kind: 1 (grab stunned enemy), kind: 3 (forced grab)\nAfter grabbing an enemy, jumps to the frame number", "Description"="Only for kind: 1 (grab stunned enemy), kind: 3 (forced grab)\nAfter grabbing an enemy, jumps to the frame number"}, "caughtact 1"={"Name"="caughtact 1", "Tip"="Only for kind: 1 (grab stunned enemy), kind: 3 (forced grab)\nAfter grabbing an enemy, the enemy's frame number jumps to the frame number", "Description"="Only for kind: 1 (grab stunned enemy), kind: 3 (forced grab)\nAfter grabbing an enemy, jumps to the frame number"}, "caughtact 2"={"Name"="caughtact 2", "Tip"="Only for kind: 1 (grab stunned enemy), kind: 3 (forced grab)\nAfter grabbing an enemy, the enemy's frame number jumps to the frame number", "Description"="Only for kind: 1 (grab stunned enemy), kind: 3 (forced grab)\nAfter grabbing an enemy, the enemy's frame number jumps to the frame number"}, "index"={"Name"="<i> index", "Tip"="injury section index", "Description"="injury section index"}}, "o"={"kind"={"Name"="kind", "Tip"="Creation type", "Description"="Creation type\n1: Dropped  \n2: Held in hand"}, "x"={"Name"="x", "Tip"="X-axis position of the object, with direction from left to right", "Description"="X-axis position of the object, with direction from left to right"}, "y"={"Name"="y", "Tip"="Y-axis position of the object, with direction from top to bottom", "Description"="Y-axis position of the object, with direction from top to bottom"}, "action"={"Name"="action", "Tip"="Frame number of the object", "Description"="Frame number of the object"}, "dvx"={"Name"="dvx", "Tip"="movement speed", "Description"="Forward (positive) and backward (negative) movement speed of the object"}, "dvy"={"Name"="dvy", "Tip"="movement speed", "Description"="Upward (negative) and downward (positive) movement speed of the object"}, "dvz"={"Name"="dvz", "Tip"="movement speed", "Description"="Vertical movement speed of the object, with direction determined by the ◆ and □ arrow keys"}, "oid"={"Name"="oid", "Tip"="Object ID", "Description"="Object ID"}, "facing"={"Name"="facing", "Tip"="Object quantity and direction", "Description"="Object quantity and direction\nOOX: OO represents the quantity. X represents the direction, where 0 = forward, 1 = reverse"}}, "c"={"kind"={"Name"="kind", "Tip"="Grab state", "Description"="1: Grabber  \n2: Grabbed"}, "x"={"Name"="x", "Tip"="X-axis position of the grabber/grabbed", "Description"="X-axis position of the grabber/grabbed"}, "y"={"Name"="y", "Tip"="Y-axis position of the grabber/grabbed", "Description"="Y-axis position of the grabber/grabbed"}, "injury"={"Name"="injury", "Tip"="Damage\nPositive value: Causes injury with hit pause effect  \nNegative value: Causes injury without hit pause effect", "Description"="Damage\nPositive value: Causes injury with hit pause effect  \nNegative value: Causes injury without hit pause effect"}, "cover"={"Name"="cover", "Tip"="Layer order\n10: Grabbed character behind  \n11: Grabbed character in front", "Description"="Layer order\n10: Grabbed character behind  \n11: Grabbed character in front"}, "vaction"={"Name"="vaction", "Tip"="Frame number of the grabbed character", "Description"="Frame number of the grabbed character"}, "aaction"={"Name"="aaction", "Tip"="When pressing Attack, jump to the corresponding frame number", "Description"="When pressing Attack, jump to the corresponding frame number"}, "taction"={"Name"="taction", "Tip"="When pressing △ + Attack, jump to the corresponding frame number", "Description"="When pressing △ + Attack, jump to the corresponding frame number"}, "hurtable"={"Name"="hurtable", "Tip"="Whether the grabbed character can be hit by others\n0: No  \n1: Yes", "Description"="Whether the grabbed character can be hit by others\n0: No  \n1: Yes"}, "decrease"={"Name"="decrease", "Tip"="Decrement value for grab duration (negative value), total duration is 301", "Description"="Decrement value for grab duration (negative value), total duration is 301"}, "fronthurtact"={"Name"="fronthurtact", "Tip"="Jump to Frame number after being hit from the front", "Description"="Jump to Frame number after being hit from the front"}, "backhurtact"={"Name"="backhurtact", "Tip"="Jump to Frame number after being hit from the back", "Description"="Jump to Frame number after being hit from the back"}, "throwvx"={"Name"="throwvx", "Tip"="X-direction speed when thrown", "Description"="X-direction speed when thrown"}, "throwvy"={"Name"="throwvy", "Tip"="Y-direction speed when thrown", "Description"="Y-direction speed when thrown"}, "throwvz"={"Name"="throwvz", "Tip"="Z-direction speed when thrown, with direction determined by the ◆ and □ arrow keys", "Description"="Z-direction speed when thrown, with direction determined by the ◆ and □ arrow keys"}, "throwinjury"={"Name"="throwinjury", "Tip"="", "Description"=""}, "dircontrol"={"Name"="dircontrol", "Tip"="", "Description"=""}}, "Other"={"File Path"={"Name"="File Path", "Tip"="", "Description"=""}, "GoTo"={"Name"="Go to Frame", "Tip"="", "Description"=""}, "Apply Change"={"Name"="Apply Change", "Tip"="", "Description"=""}, "To Next Frame"={"Name"="To Next Frame", "Tip"="", "Description"=""}}, "Menu"={"File"={"Name"="File", "Tip"="", "Description"=""}, "Open File"={"Name"="Open File", "Tip"="", "Description"=""}, "Save File"={"Name"="Save File", "Tip"="", "Description"=""}, "Exit"={"Name"="Exit", "Tip"="", "Description"=""}, "Settings"={"Name"="Settings", "Tip"="", "Description"=""}, "Preferences"={"Name"="Preferences", "Tip"="", "Description"=""}, "Help"={"Name"="Help", "Tip"="", "Description"=""}, "Show Context Help"={"Name"="Show Context Help", "Tip"="", "Description"=""}}}, "Configuration Window"={"Tab"={"Main Page"={"Name"="Main", "Tip"="", "Description"=""}, "Image Page"={"Name"="Image", "Tip"="", "Description"=""}}, "Main"={"Language"={"Name"="Language", "Tip"="", "Description"=""}, "Save"={"Name"="Save", "Tip"="", "Description"=""}, "Cancel"={"Name"="Cancel", "Tip"="", "Description"=""}}, "Path"={"Reset"={"Name"="Reset to Steam Path", "Tip"="", "Description"=""}, "Path Data"={"Name"="_res_data Folder Path", "Tip"="", "Description"=""}, "Path Png"={"Name"="_res_pngs Folder Path", "Tip"="", "Description"=""}}, "Image"={"Center Point"={"Name"={"Name"="Center Point:", "Tip"="", "Description"=""}, "Size"={"Name"="Size", "Tip"="", "Description"=""}, "Color"={"Name"="Color", "Tip"="", "Description"=""}, "Enable"={"Name"="Enable", "Tip"="", "Description"=""}}, "bp Point"={"Name"={"Name"="<bp> Point:", "Tip"="", "Description"=""}, "Size"={"Name"="Size", "Tip"="", "Description"=""}, "Color"={"Name"="Color", "Tip"="", "Description"=""}, "Enable"={"Name"="Enable", "Tip"="", "Description"=""}}, "w Point"={"Name"={"Name"="<w> Point:", "Tip"="", "Description"=""}, "Size"={"Name"="Size", "Tip"="", "Description"=""}, "Color"={"Name"="Color", "Tip"="", "Description"=""}, "Enable"={"Name"="Enable", "Tip"="", "Description"=""}}, "b Box"={"Name"={"Name"="<b> Box:", "Tip"="", "Description"=""}, "Fill Color"={"Name"="Fill Color", "Tip"="", "Description"=""}, "Border Color"={"Name"="Border Color", "Tip"="", "Description"=""}, "Enable"={"Name"="Enable", "Tip"="", "Description"=""}}, "i Box"={"Name"={"Name"="<i> Box:", "Tip"="", "Description"=""}, "Fill Color"={"Name"="Fill Color", "Tip"="", "Description"=""}, "Border Color"={"Name"="Border Color", "Tip"="", "Description"=""}, "Enable"={"Name"="Enable", "Tip"="", "Description"=""}}, "o Point"={"Name"={"Name"="<o> Point:", "Tip"="", "Description"=""}, "Size"={"Name"="Size", "Tip"="", "Description"=""}, "Color"={"Name"="Color", "Tip"="", "Description"=""}, "Enable"={"Name"="Enable", "Tip"="", "Description"=""}}, "c Point"={"Name"={"Name"="<c> Point:", "Tip"="", "Description"=""}, "Size"={"Name"="Size", "Tip"="", "Description"=""}, "Color"={"Name"="Color", "Tip"="", "Description"=""}, "Enable"={"Name"="Enable", "Tip"="", "Description"=""}}}}} ("UI Descriptions")
